vi "Retrieve from FIFO.vi"(8 "error in (no error)":errorcluster, 9 "timeout in ms (0)":i32 format="%d ms", 10 "expected iteration":u64, 11 "Transfer Group in":refnum<class "Transfer Group.lvclass">) -> (0 "error out":errorcluster, 2 "ready":bool, 3 "Transfer Group out":refnum<class "Transfer Group.lvclass">)   [LabVIEW 2017, in "DSF Core.lvlib" / "Transfer Group.lvclass"]
uses:
  Transfer Group.lvclass
  Transfer Group.lvclass/Transfer Group.ctl
  Return Timeout Error.vi
  Invalid Iteration Error.vi
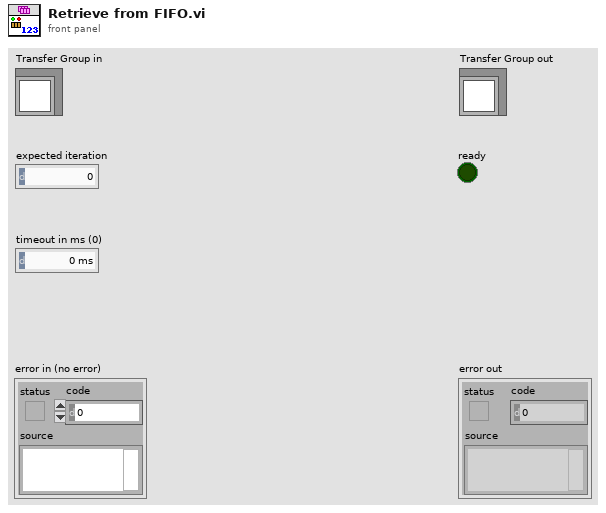
[diagram p1: front panel]
types:
  T1 = typedef "DSF Core.lvlib/DSF Timeout Behavior.ctl" = enum8{"Increment Late Count", "Throw Error"}
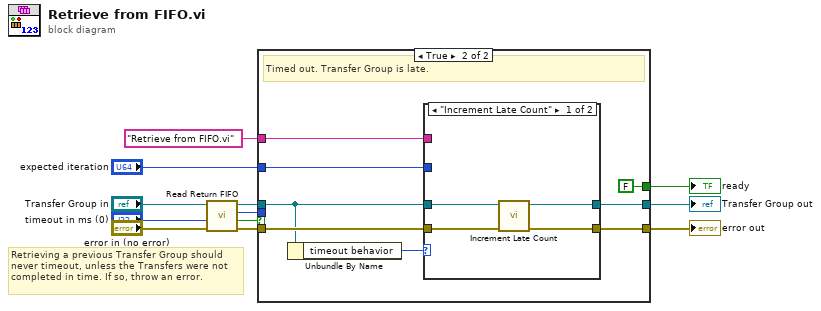
[diagram p0: block diagram]
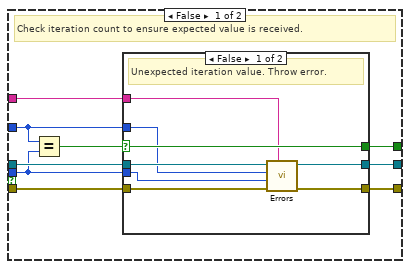
[diagram p2: hidden frame]
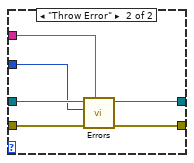
[diagram p4: hidden frame]
diagram:
  # "Retrieving a previous Transfer Group should never timeout, unless the Transfers were not completed in time. If so, throw an error."
  n1 = call "Read Return FIFO.vi"("error in (no error)"="error in (no error)", "timeout in ms (0)"="timeout in ms (0)", "Transfer Group in"="Transfer Group in") -> ("error out"=w12:errorcluster, "timed out?"=w11:bool, "Transfer Group iteration"=w9:u64, "Transfer Group out"=w10:refnum<class "Transfer Group.lvclass">)  [unwired: 5 in]
  n2 = case shown="True" w11 {
    tunnel: w12 -> [w18 w39]
    tunnel: w10 -> [w20 w35]
    tunnel: w9 -> [w14 _]
    tunnel: "expected iteration" -> [w13 w34]
    tunnel: [w17 w36] -> w2
    tunnel: [w19 w37] -> w1
    tunnel: [w16 FALSE] -> w5
    tunnel: "Retrieve from FIFO.vi" ("error source vi name") -> [w15 w38]
    frame False {
      # "Check iteration count to ensure expected value is received."
      n3 = Equal?(x=w13, y=w14) -> (x = y?=w21:bool)
      n4 = case shown="False" w21 {
        selector: w21 -> [w29 w30]
        tunnel: w20 -> [w28 w32]
        tunnel: [w26 w32] -> w19
        tunnel: w18 -> [w27 w31]
        tunnel: [w25 w31] -> w17
        tunnel: [w29 w30] -> w16
        tunnel: w15 -> [w24 _]
        tunnel: w14 -> [w22 _]
        tunnel: w13 -> [w23 _]
        frame False {
          # "Unexpected iteration value. Throw error."
          n5 = call-poly "Errors.vi"("error source vi name"=w24, "error in (no error)"=w27, "actual iteration"=w22, "expected iteration"=w23, "Transfer Group in"=w28) -> ("error out"=w25:errorcluster, "Transfer Group out"=w26:refnum<class "Transfer Group.lvclass">)  [unwired: 5 in]
        }
        frame True {
          # "Expected value. Proceed."
        }
      }
    }
    frame True {
      # "Timed out. Transfer Group is late."
      n6 = Unbundle By Name(w35) -> ("timeout behavior"=w33:T1)
      n7 = case shown="\"Increment Late Count\"" w33 {
        tunnel: w39 -> [w43 w50]
        tunnel: w38 -> [_ w49]
        tunnel: [w41 w48] -> w37
        tunnel: [w42 w47] -> w36
        tunnel: w35 -> [w44 w46]
        tunnel: w34 -> [_ w45]
        frame "Increment Late Count" {
          n8 = call "Increment Late Count.vi"("error in (no error)"=w43, "Transfer Group in"=w44) -> ("error out"=w42:errorcluster, "Transfer Group out"=w41:refnum<class "Transfer Group.lvclass">)  [unwired: 8 in]
        }
        frame "Throw Error" {
          n9 = call-poly "Errors.vi"("error source vi name"=w49, "error in (no error)"=w50, "expected iteration"=w45, "Transfer Group in"=w46) -> ("error out"=w47:errorcluster, "Transfer Group out"=w48:refnum<class "Transfer Group.lvclass">)  [unwired: 6 in]
        }
      }
    }
  }
  "error out" <- w2
  "Transfer Group out" <- w1
  "ready" <- w5
